vi "WaveformBuffer_SubVI.vi"(11 "Main Data Cluster in":T1={"Notes Frequency Array"=[], "Main Waveform Type"=enum."Sine", "Waveform"={"t0"=timestamp(0 s since 1904-01-01), "dt"=1.0, "Y"=[]}, "Main Current Note"=0, "Octave Range Offset"=0, "sound format"={"sample rate (S/s)"=22050.0, "number of channels"=2, "bits per sample"=16}, "Task ID"=0, "Note Duration"=0.0, "Volume"=0.0, "ADSR Envelope Cluster"={"Decay"=0, "Sustain"=0, "Attack"=0, "Release"=0}, "Playing?"=FALSE, "Pitch LFO"={"Rate"=0.0, "Ammount"=0.0}, "device ID"=0, "Filter Section"={"Lowpass Freq"=0.0, "Highpass Freq"=0.0, "Enable"=FALSE}, "Distortion"={"Distortion level"=0.0, "Enable"=FALSE}, "Secondary Waveform Type"=enum."Sine", "Secondary Frequency"=0.0, "Secondary Blend"=0.0, "Envelope XY Graph"={[], []}, "Buffer Number"=0, "End of Sequence?"=FALSE} {"task ID" format="%.0x"}) -> (2 "waveform out":waveform(dbl), 3 "Main Data Cluster out":T1={"Notes Frequency Array"=[], "Main Waveform Type"=enum."Sine", "Waveform"={"t0"=timestamp(0 s since 1904-01-01), "dt"=1.0, "Y"=[]}, "Main Current Note"=0, "Octave Range Offset"=0, "sound format"={"sample rate (S/s)"=22050.0, "number of channels"=2, "bits per sample"=16}, "Task ID"=0, "Note Duration"=0.0, "Volume"=0.0, "ADSR Envelope Cluster"={"Decay"=0, "Sustain"=0, "Attack"=0, "Release"=0}, "Playing?"=FALSE, "Pitch LFO"={"Rate"=0.0, "Ammount"=0.0}, "device ID"=0, "Filter Section"={"Lowpass Freq"=0.0, "Highpass Freq"=0.0, "Enable"=FALSE}, "Distortion"={"Distortion level"=0.0, "Enable"=FALSE}, "Secondary Waveform Type"=enum."Sine", "Secondary Frequency"=0.0, "Secondary Blend"=0.0, "Envelope XY Graph"={[], []}, "Buffer Number"=0, "End of Sequence?"=FALSE} {"task ID" format="%.0x"})   [LabVIEW 2024]
doc: "This SubVI creates a buffer of 128 (variable number) samples with built it mechanics of a ring counter for the notes in a sequence.\n\nIN: Main Data Cluster in;\nOUT: Main Data Cluster out; waveform out;"
uses:
  controls/#typedef_Waveform_Type.ctl
  <vilib>/sound2/lvsound2.llb/Sound Data Format.ctl
  <vilib>/sound2/lvsound2.llb/Sound Output Task ID.ctl
  controls/#typedef_Data_Cluster.ctl
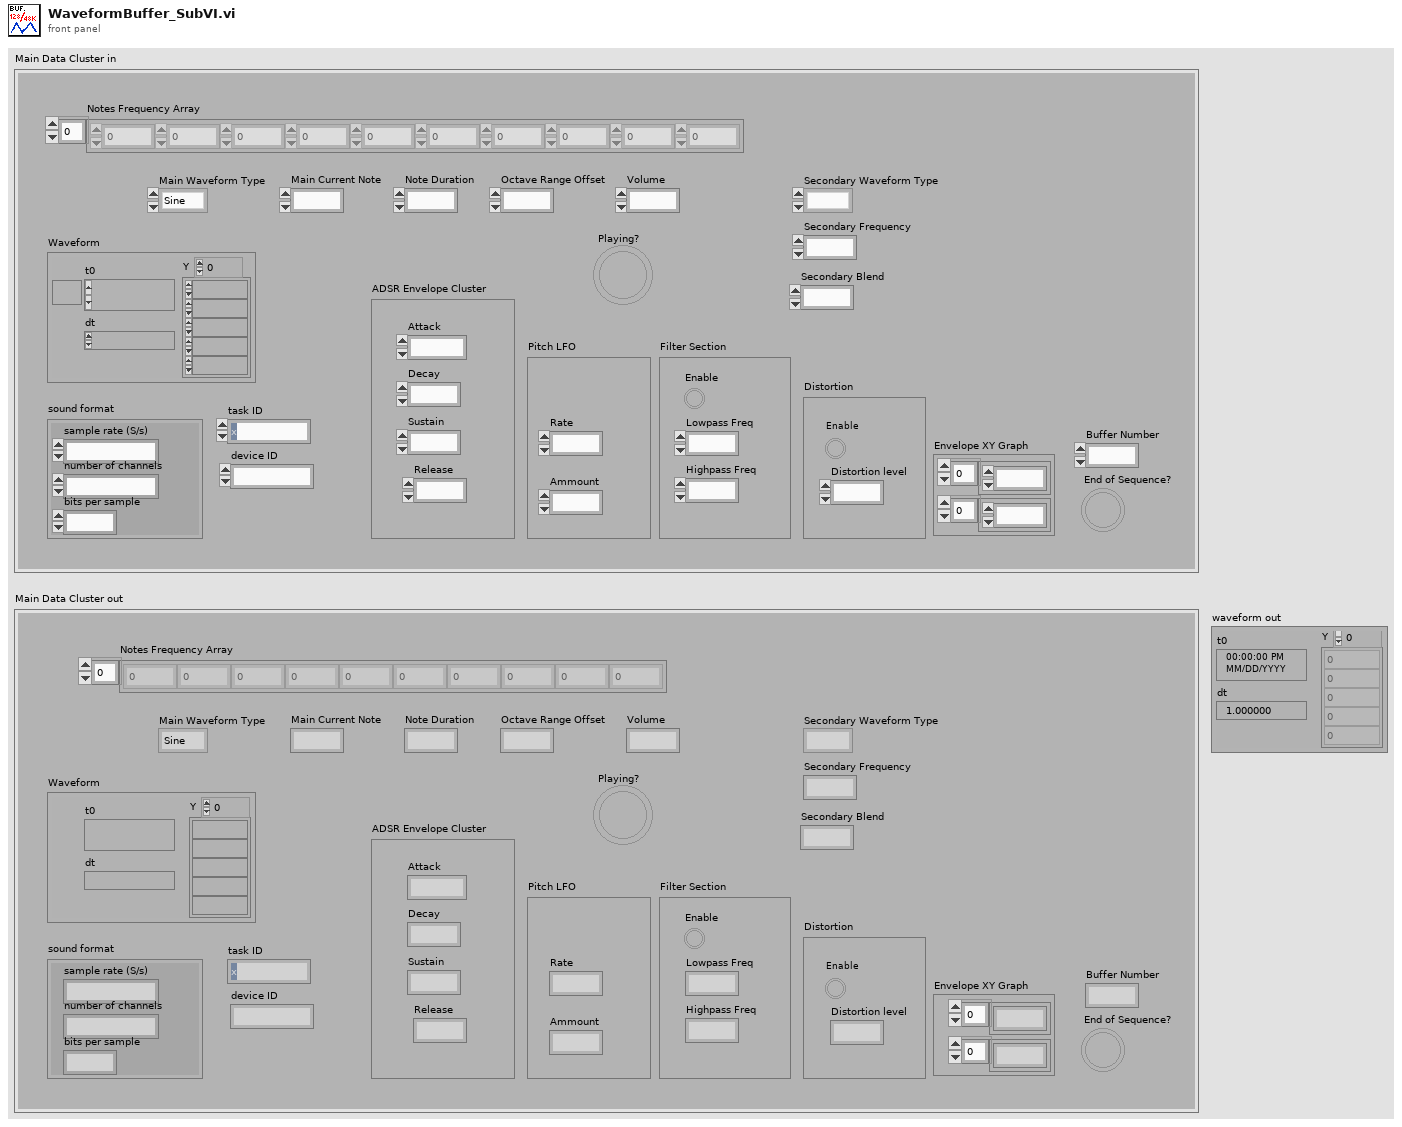
[diagram p1: front panel]
types:
  T1 = typedef "#typedef_Data_Cluster.ctl" = cluster{"Notes Frequency Array":dbl[], "Main Waveform Type":T2, "Waveform":waveform(dbl), "Main Current Note":i32, "Octave Range Offset":u32, "sound format":T3, "Task ID":T4, "Note Duration":dbl, "Volume":dbl, "ADSR Envelope Cluster":cluster{"Decay":i32, "Sustain":i32, "Attack":i32, "Release":i32}, "Playing?":bool, "Pitch LFO":cluster{"Rate":dbl, "Ammount":dbl}, "device ID":u32, "Filter Section":cluster{"Lowpass Freq":dbl, "Highpass Freq":dbl, "Enable":bool}, "Distortion":cluster{"Distortion level":dbl, "Enable":bool}, "Secondary Waveform Type":T2, "Secondary Frequency":dbl, "Secondary Blend":dbl, "Envelope XY Graph":cluster{dbl[], dbl[]}, "Buffer Number":i32, "End of Sequence?":bool}
  T2 = typedef "#typedef_Waveform_Type.ctl" = enum16{"Sine", "Saw", "Square", "Triangle", "Noise"}
  T3 = typedef "Sound Data Format.ctl" = cluster{"sample rate (S/s)":dbl, "number of channels":i32, "bits per sample":i32}
  T4 = typedef "Sound Output Task ID.ctl" = u32
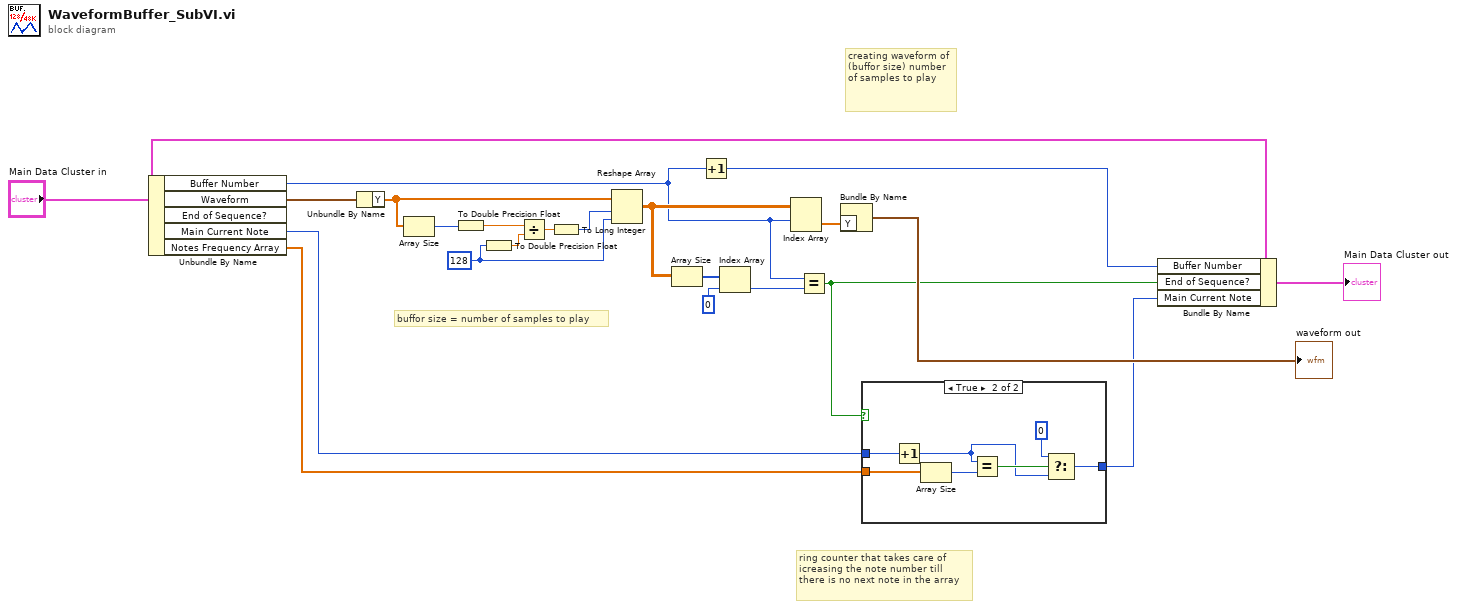
[diagram p0: block diagram]
diagram:
  w6 = 128 ("y")
  # "creating waveform of (buffor size) number of samples to play"
  # "ring counter that takes care of icreasing the note number till there is no next note in the array"
  # "buffor size = number of samples to play"
  n1 = Unbundle By Name("Main Data Cluster in") -> ("Buffer Number"=w5:i32, "Waveform"=w17:waveform(dbl), "Main Current Note"=w3:i32, "Notes Frequency Array"=w4:dbl[])  [unwired: 1 out]
  n2 = Unbundle By Name(w17) -> ("Y"=w18:dbl[])
  n3 = Array Size(array=w18) -> (size(s)=w19:i32)
  n4 = To Double Precision Float(number=w19) -> (double precision float=w14:dbl)
  n5 = To Double Precision Float(number=w6) -> (double precision float=w13:dbl)
  n6 = Divide(x=w14, y=w13) -> (x/y=w20:dbl)
  n7 = To Long Integer(number=w20) -> (32bit integer=w12:i32)
  n8 = Reshape Array(w18, w12, w6) -> (w22:dbl[][])
  n9 = Array Size(array=w22) -> (size(s)=w10:i32[])
  n10 = Increment(x=w5) -> (x+1=w15:i32)
  n11 = Index Array(array=w10, index=0) -> (element=w9:i32)
  n12 = Index Array(array=w22, index (row)=w5) -> (element=w21:dbl[])  [unwired: 1 in]
  n13 = Equal?(x=w5, y=w9) -> (x = y?=w2:bool)
  n14 = Bundle By Name("Y"=w21) -> (→"waveform out":waveform(dbl))  [unwired: 1 in]
  n15 = case shown="True" w2 {
    tunnel: w4 -> [_ w30]
    tunnel: w3 -> [w23 w26]
    tunnel: [w23 w24] -> w1
    frame False {
    }
    frame True {
      n16 = Increment(x=w26) -> (x+1=w28:i32)
      n17 = Array Size(array=w30) -> (size(s)=w25:i32)
      n18 = Equal?(x=w28, y=w25) -> (x = y?=w29:bool)
      n19 = Select(t=0, s=w29, f=w28) -> (s? t:f=w24:i32)
    }
  }
  n20 = Bundle By Name(cluster="Main Data Cluster in", "Buffer Number"=w15, "End of Sequence?"=w2, "Main Current Note"=w1) -> (→"Main Data Cluster out":T1)
